vi "CloseVeriStandConnection.vi"(8 "error in (no error)":errorcluster, 11 "VeriStand Test Case in":refnum<class "VeriStandTestCase.lvclass">) -> (0 "error out":errorcluster, 3 "VeriStand Test Case out":refnum<class "VeriStandTestCase.lvclass">)   [LabVIEW 2027, in "VeriStandTestCase.lvclass"]
uses:
  VeriStandTestCase.lvclass
  VeriStandTestCase.lvclass/VeriStandTestCase.ctl
  <vilib>/NI VeriStand/Execution/Workspace/NI_VS Workspace ExecutionAPI.lvlib
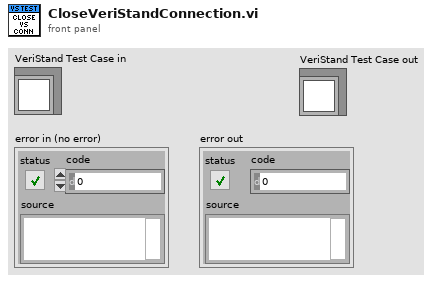
[diagram p1: front panel]
types:
  T1 = typedef "NI_VS Workspace ExecutionAPI.lvlib/WorkspaceAPI.ctl" = refnum<k39>
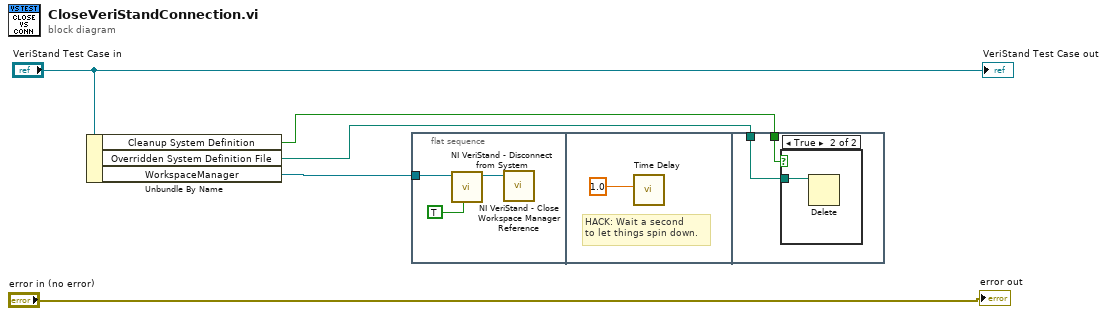
[diagram p0: block diagram]
diagram:
  n1 = Unbundle By Name("VeriStand Test Case in") -> ("Cleanup System Definition"=w1:bool, "Overridden System Definition File"=w2:path, "WorkspaceManager"=w5:T1)
  n2 = flat-sequence {
    tunnel: w5 -> [w7]
    tunnel: w2 -> [w11]
    tunnel: w1 -> [w10]
    frame #0 {
      n3 = call <vilib>:"NI VeriStand - Disconnect from System.vi"("Undeploy System Definition (F)"=TRUE, "WorkspaceManager in"=w7) -> ("WorkspaceManager out"=w6:T1)  [unwired: 8 in, 1 out]
      n4 = call <vilib>:"NI VeriStand - Close Workspace Manager Reference.vi"("WorkspaceManager"=w6) -> ()  [unwired: 10 in, 1 out]
    }
    frame #1 {
      # "HACK: Wait a second\nto let things spin down."
      n5 = call "Time Delay"("Delay Time (s)"=1.0) -> ()  [unwired: 10 in, 1 out]
    }
    frame #2 {
      n6 = case shown="True" w10 {
        tunnel: w11 -> [_ w12]
        frame False {
        }
        frame True {
          n7 = Delete(path (use dialog)=w12) -> ()  [unwired: 4 in, 3 out]
        }
      }
    }
  }
  "error out" <- "error in (no error)"
  "VeriStand Test Case out" <- "VeriStand Test Case in"
